vi "Serial Channel Output.vi"(0 "tagged llp packets cluster":T1, 1 "reset":bool, 2 "global counter":T25, 3 "common resources":T11={"sync pulse resources"={"sync pulse destination terminal"="", "sync100"="", "sync pulse source terminal"="", "imported sync pulse register"="", "generate sync pulse handshake"="", "enable sync pulse register"="", "sync pulse clock"=""}, "serial channel resources"={"sc 0"={"completed frames register"=""}, "sc 1"={"completed frames register"=""}, "sc 2"={"completed frames register"=""}, "sc 3"={"completed frames register"=""}, "sc 4"={"completed frames register"=""}, "sc 5"={"completed frames register"=""}, "sc 6"={"completed frames register"=""}, "sc 7"={"completed frames register"=""}}, "dram manager 0"={"DRAM class"=refnum, "process clock"="", "registers"={"configuration"={"write time slice"="", "request time slice"="", "DRAM arbiter config"="", "partition config"=""}, "reset"={"handshake"={"start.go"="", "start.go rcvd"="", "done.go"="", "done.go rcvd"=""}, "process"={"in"="", "out"=""}, "write"={"in"="", "out 0"="", "out 1"="", "out 2"="", "out 3"=""}, "read"={"in"="", "out 0"="", "out 1"="", "out 2"="", "out 3"=""}}, "status"={"partition full"=""}}, "FIFOs"={"write data"={"FIFO 0"="", "FIFO 1"="", "FIFO 2"="", "FIFO 3"=""}, "request metadata"={"FIFO"=""}, "read data VOQ"={"FIFO 0"="", "FIFO 1"="", "FIFO 2"="", "FIFO 3"=""}, "read data"={"FIFO 0"="", "FIFO 1"="", "FIFO 2"="", "FIFO 3"=""}}, "num active streams"=0.0, "max open read requests"=256}, "dram manager 1"={"DRAM class"=refnum, "process clock"="", "registers"={"configuration"={"write time slice"="", "request time slice"="", "DRAM arbiter config"="", "partition config"=""}, "reset"={"handshake"={"start.go"="", "start.go rcvd"="", "done.go"="", "done.go rcvd"=""}, "process"={"in"="", "out"=""}, "write"={"in"="", "out 0"="", "out 1"="", "out 2"="", "out 3"=""}, "read"={"in"="", "out 0"="", "out 1"="", "out 2"="", "out 3"=""}}, "status"={"partition full"=""}}, "FIFOs"={"write data"={"FIFO 0"="", "FIFO 1"="", "FIFO 2"="", "FIFO 3"=""}, "request metadata"={"FIFO"=""}, "read data VOQ"={"FIFO 0"="", "FIFO 1"="", "FIFO 2"="", "FIFO 3"=""}, "read data"={"FIFO 0"="", "FIFO 1"="", "FIFO 2"="", "FIFO 3"=""}}, "num active streams"=0.0, "max open read requests"=256}}, 5 "dram status":T22[](array[typedef]), 7 "start trigger":bool, 9 "output valid":bool[](array[boolean])=[FALSE, FALSE, FALSE, FALSE, FALSE, FALSE, FALSE, FALSE], 11 "stop trigger":bool, 12 "channel configs":T24[](array[typedef])) -> (4 "serial output channel status":T26[](array[typedef]), 6 "ready for start trigger":bool, 8 "packet timing error detected":bool, 10 "generation done":bool, 14 "ready for input":bool[](array[boolean]), 15 "i2c monitor array":T23[](array[typedef]) {"monitor word" format="%.0x"})   [LabVIEW 2020, in "GettingStarted_Gen_148X_FPGA.lvlib"]
uses:
  GettingStarted_Gen_148X_FPGA.lvlib
  Types/Serial Output Channel Status.ctl
  Common/Types/DRAM Status.ctl
  <instrlib>/FlexRIO/CSI-2/v2/FPGA/Types/Timestamp Counter Value.ctl
  Types/Serial Output Channel Datapath Configuration.ctl
  <instrlib>/FlexRIO/API/FPGA/v1/IO/NI148x/i2c monitor.ctl
  Common/Types/Common Resources.ctl
  <instrlib>/_niInstr/Memory/v1/FPGA/DRAM/niInstr Memory DRAM v1 FPGA.lvclass
  <instrlib>/FlexRIO/CSI-2/v2/FPGA/Types/Sync Pulse Resources.ctl
  Common/Types/Serial Channel Resources.ctl
  Common/Types/Single Serial Channel Resources.ctl
  <instrlib>/FlexRIO/CSI-2/v2/FPGA/DRAM Manager/Private/DRAM Manager.ctl
  <instrlib>/FlexRIO/CSI-2/v2/FPGA/DRAM Manager/Private/Common/DRAM Manager Registers.ctl
  <instrlib>/FlexRIO/CSI-2/v2/FPGA/DRAM Manager/Private/Common/Handshake Registers.ctl
  <instrlib>/FlexRIO/CSI-2/v2/FPGA/DRAM Manager/Private/Common/DRAM Manager FIFOs.ctl
  <instrlib>/FlexRIO/CSI-2/v2/FPGA/DRAM Manager/Private/Common/Write Data FIFO Ref.ctl
  <instrlib>/FlexRIO/CSI-2/v2/FPGA/DRAM Manager/Private/Common/Read Request Metadata FIFO Ref.ctl
  <instrlib>/FlexRIO/CSI-2/v2/FPGA/DRAM Manager/Private/Common/Read Data FIFO Ref.ctl
  Common/Types/Tagged LLP Packets Cluster.ctl
  <instrlib>/FlexRIO/CSI-2/v2/FPGA/Types/Tagged LLP Packet.ctl
  <instrlib>/FlexRIO/CSI-2/v2/FPGA/Types/FPGA LLP Packet Tag.ctl
  <instrlib>/FlexRIO/CSI-2/v2/FPGA/Types/FPGA LLP Packet Timestamp.ctl
  <instrlib>/FlexRIO/CSI-2/v2/FPGA/Types/Timestamp ID.ctl
  <instrlib>/FlexRIO/CSI-2/v2/FPGA/Types/FPGA LLP Packet Size.ctl
  <instrlib>/FlexRIO/CSI-2/v2/FPGA/Types/LLP Packet.ctl
  <instrlib>/FlexRIO/CSI-2/v2/FPGA/Types/LLP Packet Header.ctl
  <instrlib>/FlexRIO/CSI-2/v2/FPGA/Types/LLP Packet Payload.ctl
  <instrlib>/FlexRIO/CSI-2/v2/FPGA/Types/LLP Packet Footer.ctl
  Common/GettingStarted_Common_148X_FPGA.lvlib
  <instrlib>/_niInstr/Basic Elements/v1/FPGA/niInstr Basic Elements v1 FPGA.lvlib
  <instrlib>/FlexRIO/CSI-2/v2/FPGA/NI CSI-2 API FPGA v2.lvlib
  <instrlib>/FlexRIO/API/FPGA/v1/IO/NI148x/FlexRIO 148x FPGA v1.lvlib
  <instrlib>/FlexRIO/CSI-2/v2/FPGA/DRAM Manager/DRAM Manager v2.lvlib
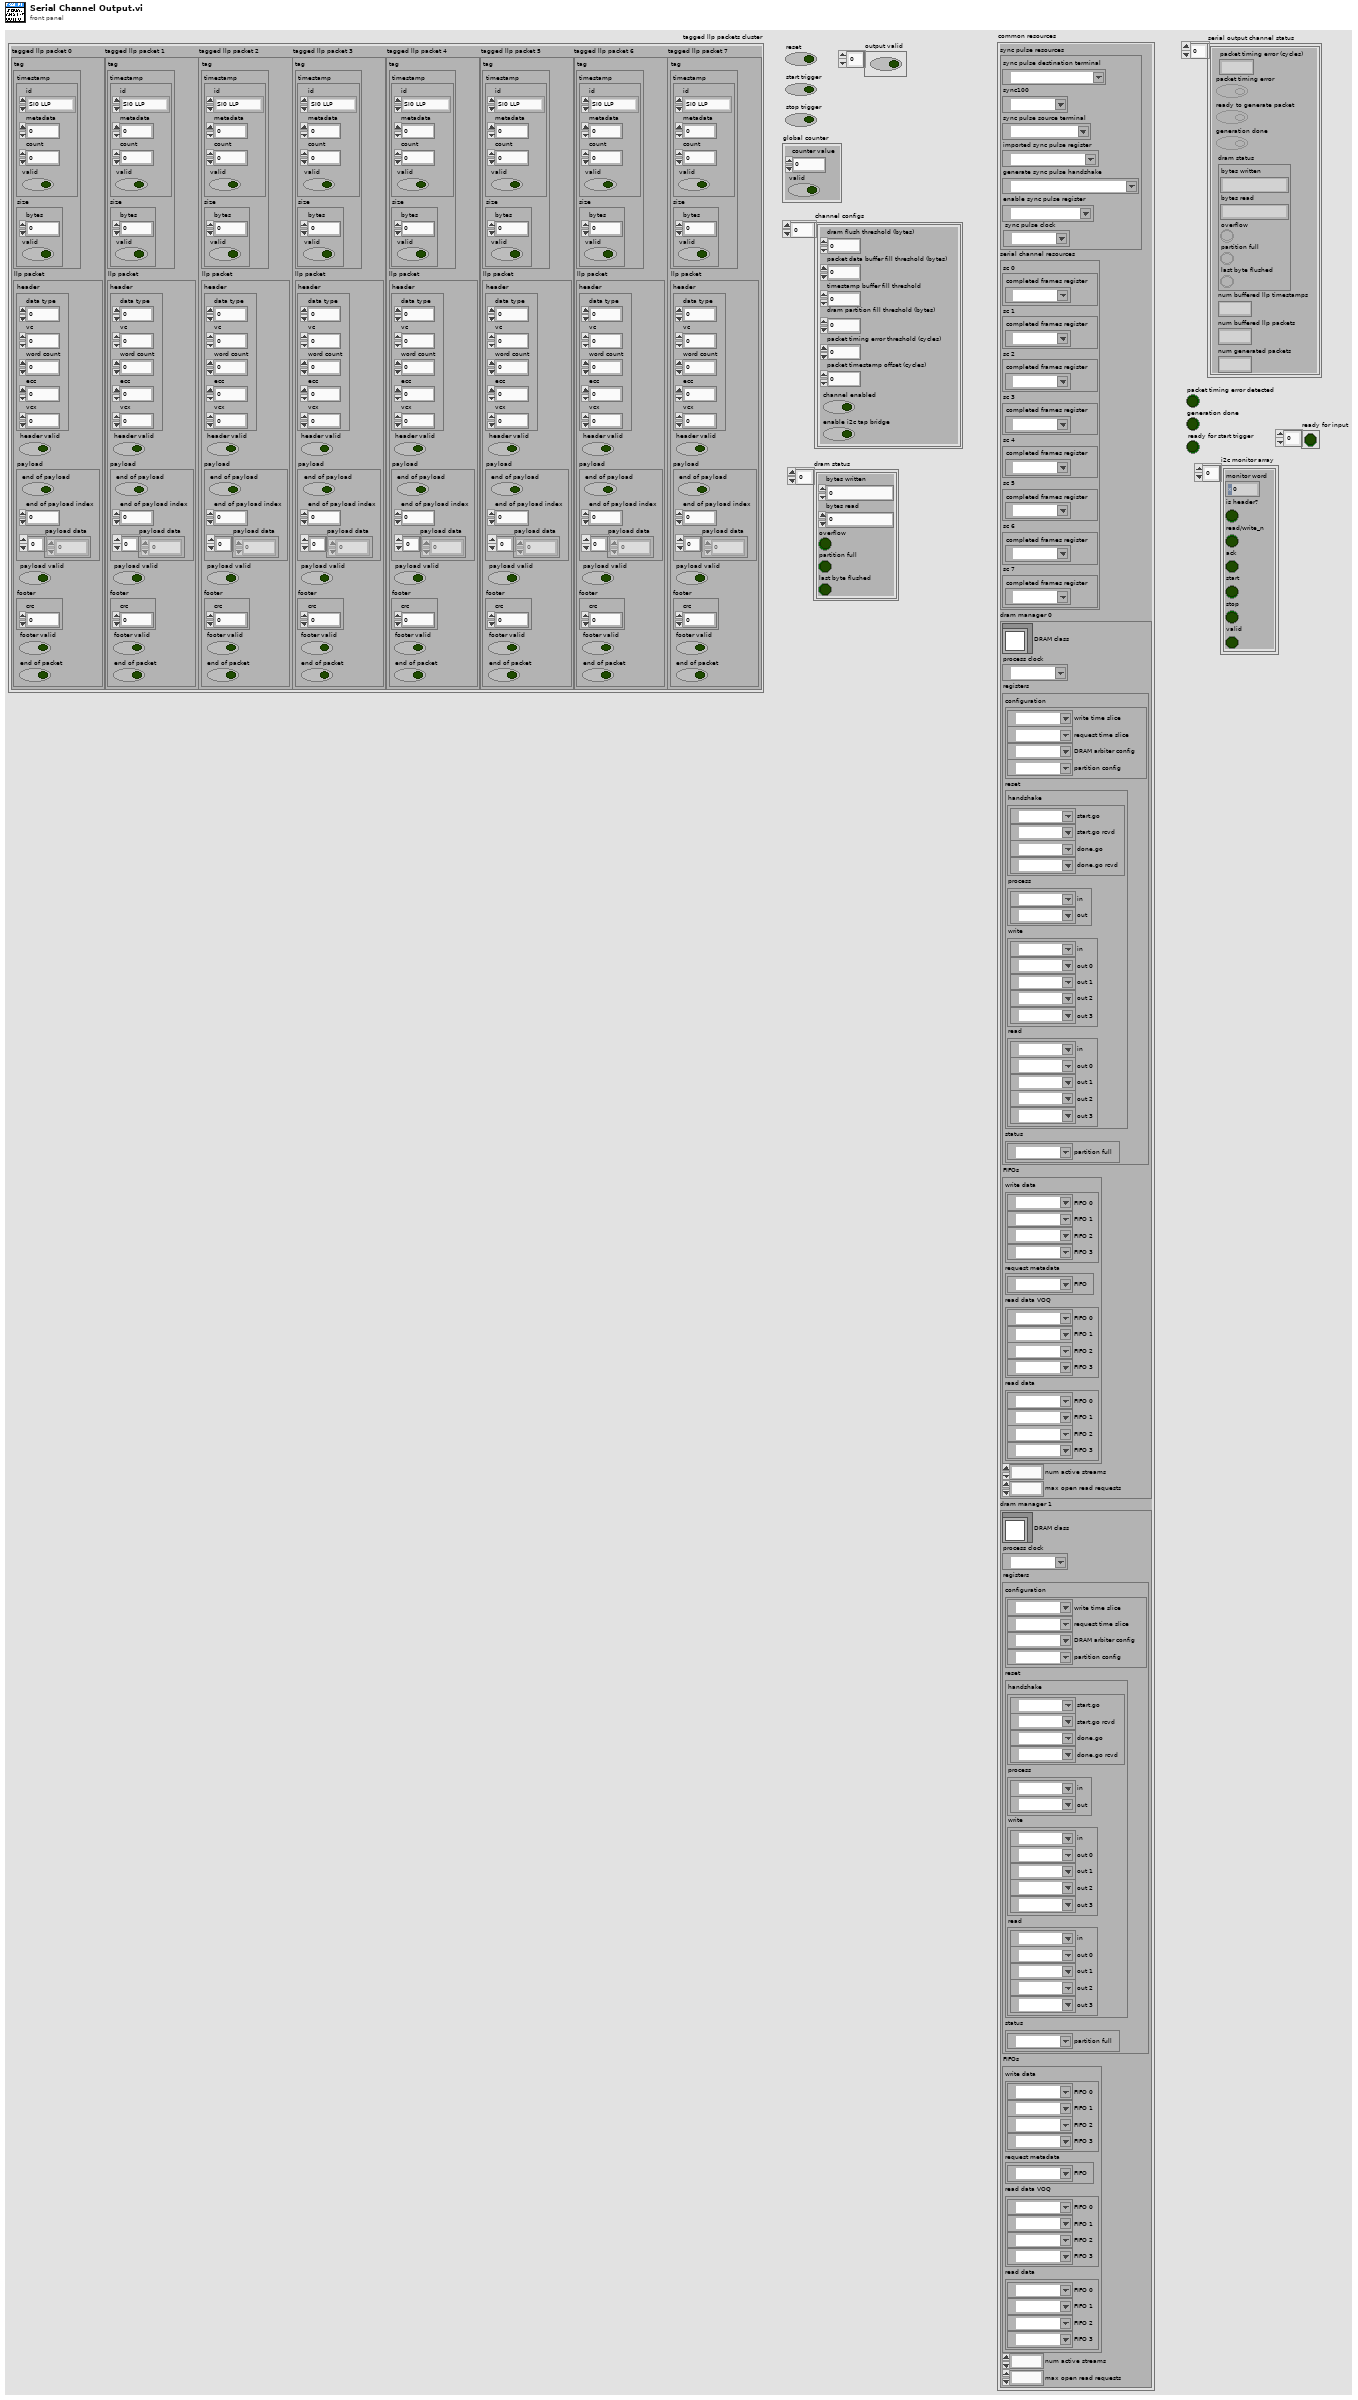
[diagram p1: front panel]
types:
  T1 = typedef "GettingStarted_Common_148X_FPGA.lvlib/Tagged LLP Packets Cluster.ctl" = cluster{"tagged llp packet 0":T2, "tagged llp packet 1":T2, "tagged llp packet 2":T2, "tagged llp packet 3":T2, "tagged llp packet 4":T2, "tagged llp packet 5":T2, "tagged llp packet 6":T2, "tagged llp packet 7":T2}
  T2 = typedef "NI CSI-2 API FPGA v2.lvlib/Tagged LLP Packet.ctl" = cluster{"tag":T3, "llp packet":T7}
  T3 = typedef "NI CSI-2 API FPGA v2.lvlib/FPGA LLP Packet Tag.ctl" = cluster{"timestamp":T4, "size":T6}
  T4 = typedef "NI CSI-2 API FPGA v2.lvlib/FPGA LLP Packet Timestamp.ctl" = cluster{"valid":bool, "count":fxp<+,50,50>, "id":T5, "metadata":u8}
  T5 = typedef "NI CSI-2 API FPGA v2.lvlib/Timestamp ID.ctl" = enum8{"SI0 LLP", "SI1 LLP", "SI2 LLP", "SI3 LLP", "SI4 LLP", "SI5 LLP", "SI6 LLP", "SI7 LLP", "SO0 LLP", "SO1 LLP", "SO2 LLP", "SO3 LLP", "SO4 LLP", "SO5 LLP", "SO6 LLP", "SO7 LLP", "Ser0 GPIO Bank", "Ser1 GPIO Bank", "Ser2 GPIO Bank", "Ser3 GPIO Bank", "Ser4 GPIO Bank", "Ser5 GPIO Bank", "Ser6 GPIO Bank", "Ser7 GPIO Bank", "Des0 GPIO Bank", "Des1 GPIO Bank", "Des2 GPIO Bank", "Des3 GPIO Bank", "Des4 GPIO Bank", "Des5 GPIO Bank", "Des6 GPIO Bank", "Des7 GPIO Bank", "User0", "User1", "User2", "User3", "User4", "User5", "User6", "User7", "User8", "User9", "User10", "User11", "User12", "User13", "User14", "User15", "User16", "User17", "User18", "User19", "User20", "User21", "User22", "User23", "User24", "User25", "User26", "User27", "User28", "User29", "User30", "User31"}
  T6 = typedef "NI CSI-2 API FPGA v2.lvlib/FPGA LLP Packet Size.ctl" = cluster{"bytes":fxp<+,17,17>, "valid":bool}
  T7 = typedef "NI CSI-2 API FPGA v2.lvlib/LLP Packet.ctl" = cluster{"header":T8, "header valid":bool, "payload":T9, "payload valid":bool, "footer":T10, "footer valid":bool, "end of packet":bool}
  T8 = typedef "NI CSI-2 API FPGA v2.lvlib/LLP Packet Header.ctl" = cluster{"word count":u16, "ecc":fxp<+,6,6>, "vcx":fxp<+,2,2>, "data type":fxp<+,6,6>, "vc":fxp<+,2,2>}
  T9 = typedef "NI CSI-2 API FPGA v2.lvlib/LLP Packet Payload.ctl" = cluster{"end of payload":bool, "end of payload index":fxp<+,3,3>, "payload data":u8[]}
  T10 = typedef "NI CSI-2 API FPGA v2.lvlib/LLP Packet Footer.ctl" = cluster{"crc":u16}
  T11 = typedef "GettingStarted_Common_148X_FPGA.lvlib/Common Resources.ctl" = cluster{"sync pulse resources":T12, "serial channel resources":T13, "dram manager 0":T15, "dram manager 1":T15}
  T12 = typedef "NI CSI-2 API FPGA v2.lvlib/Sync Pulse Resources.ctl" = cluster{"sync pulse destination terminal":refnum<k21>, "sync100":refnum<k21>, "sync pulse source terminal":refnum<k21>, "imported sync pulse register":refnum<k21>, "generate sync pulse handshake":refnum<k21>, "enable sync pulse register":refnum<k21>, "sync pulse clock":refnum<k21>}
  T13 = typedef "GettingStarted_Common_148X_FPGA.lvlib/Serial Channel Resources.ctl" = cluster{"sc 0":T14, "sc 1":T14, "sc 2":T14, "sc 3":T14, "sc 4":T14, "sc 5":T14, "sc 6":T14, "sc 7":T14}
  T14 = typedef "GettingStarted_Common_148X_FPGA.lvlib/Single Serial Channel Resources.ctl" = cluster{"completed frames register":refnum<k21>}
  T15 = typedef "DRAM Manager v2.lvlib/DRAM Manager.ctl" = cluster{"DRAM class":refnum<class "niInstr Memory DRAM v1 FPGA.lvclass">, "process clock":refnum<k21>, "registers":T16, "FIFOs":T18, "num active streams":fxp<+,3,3>, "max open read requests":u16}
  T16 = typedef "DRAM Manager v2.lvlib/DRAM Manager Registers.ctl" = cluster{"configuration":cluster{"write time slice":refnum<k21>, "request time slice":refnum<k21>, "DRAM arbiter config":refnum<k21>, "partition config":refnum<k21>}, "reset":cluster{"handshake":T17, "process":cluster{"in":refnum<k21>, "out":refnum<k21>}, "write":cluster{"in":refnum<k21>, "out 0":refnum<k21>, "out 1":refnum<k21>, "out 2":refnum<k21>, "out 3":refnum<k21>}, "read":cluster{"in":refnum<k21>, "out 0":refnum<k21>, "out 1":refnum<k21>, "out 2":refnum<k21>, "out 3":refnum<k21>}}, "status":cluster{"partition full":refnum<k21>}}
  T17 = typedef "DRAM Manager v2.lvlib/Handshake Registers.ctl" = cluster{"start.go":refnum<k21>, "start.go rcvd":refnum<k21>, "done.go":refnum<k21>, "done.go rcvd":refnum<k21>}
  T18 = typedef "DRAM Manager v2.lvlib/DRAM Manager FIFOs.ctl" = cluster{"write data":cluster{"FIFO 0":T19, "FIFO 1":T19, "FIFO 2":T19, "FIFO 3":T19}, "request metadata":cluster{"FIFO":T20}, "read data VOQ":cluster{"FIFO 0":T21, "FIFO 1":T21, "FIFO 2":T21, "FIFO 3":T21}, "read data":cluster{"FIFO 0":T21, "FIFO 1":T21, "FIFO 2":T21, "FIFO 3":T21}}
  T19 = typedef "DRAM Manager v2.lvlib/Write Data FIFO Ref.ctl" = refnum<k21>
  T20 = typedef "DRAM Manager v2.lvlib/Read Request Metadata FIFO Ref.ctl" = refnum<k21>
  T21 = typedef "DRAM Manager v2.lvlib/Read Data FIFO Ref.ctl" = refnum<k21>
  T22 = typedef "GettingStarted_Common_148X_FPGA.lvlib/DRAM Status.ctl" = cluster{"bytes written":u64, "bytes read":u64, "overflow":bool, "partition full":bool, "last byte flushed":bool}
  T23 = typedef "FlexRIO 148x FPGA v1.lvlib/i2c monitor.ctl" = cluster{"monitor word":u8, "is header?":bool, "read/write_n":bool, "ack":bool, "start":bool, "stop":bool, "valid":bool}
  T24 = typedef "GettingStarted_Gen_148X_FPGA.lvlib/Serial Output Channel Datapath Configuration.ctl" = cluster{"dram flush threshold (bytes)":u64, "packet data buffer fill threshold (bytes)":u64, "timestamp buffer fill threshold":u32, "packet timing error threshold (cycles)":u64, "channel enabled":bool, "dram partition fill threshold (bytes)":u64, "enable i2c tap bridge":bool, "packet timestamp offset (cycles)":i64}
  T25 = typedef "NI CSI-2 API FPGA v2.lvlib/Timestamp Counter Value.ctl" = cluster{"counter value":u64, "valid":bool}
  T26 = typedef "GettingStarted_Gen_148X_FPGA.lvlib/Serial Output Channel Status.ctl" = cluster{"num buffered llp packets":fxp<+,14,14>, "packet timing error (cycles)":u64, "packet timing error":bool, "ready to generate packet":bool, "dram status":T22, "num buffered llp timestamps":u32, "generation done":bool, "num generated packets":u64}
  T27 = cluster{"datapath configs":T24, "tagged llp packet":T2, "output valid":bool, "dram status":T22}
  T28 = typedef "GettingStarted_Gen_148X_FPGA.lvlib/8 Out Channel Resources.ctl" = cluster{"so 0 resources":T29, "so 1 resources":T29, "so 2 resources":T29, "so 3 resources":T29, "so 4 resources":T29, "so 5 resources":T29, "so 6 resources":T29, "so 7 resources":T29}
  T29 = typedef "GettingStarted_Gen_148X_FPGA.lvlib/Serial Output Channel Resources.ctl" = cluster{"csi-2 output io":T30, "serial output channel instance":u8, "i2c io":T31, "sc resources":T14}
  T30 = typedef "GettingStarted_Common_148X_FPGA.lvlib/Serial Output Channel IO.ctl" = cluster{"csi-2 axi stream tdata":refnum<k21>, "csi-2 axi stream tlast":refnum<k21>, "csi-2 axi stream tvalid":refnum<k21>, "csi-2 axi stream tuser":refnum<k21>, "csi-2 axi stream tready":refnum<k21>, "num packets in tx fifo":refnum<k21>, "ready to transmit packet":refnum<k21>, "transmit packet done":refnum<k21>, "transmit packet":refnum<k21>}
  T31 = typedef "GettingStarted_Common_148X_FPGA.lvlib/I2C IO.ctl" = cluster{"sda input":refnum<k21>, "sda output enable":refnum<k21>, "scl input":refnum<k21>, "scl output enable":refnum<k21>}
  T32 = typedef "GettingStarted_Gen_148X_FPGA.lvlib/4 In 4 Out Channel Resources.ctl" = cluster{"so 0 resources":T29, "so 1 resources":T29, "so 2 resources":T29, "so 3 resources":T29, "si 0 resources":T33, "si 1 resources":T33, "si 2 resources":T33, "si 3 resources":T33}
  T33 = typedef "GettingStarted_Gen_148X_FPGA.lvlib/Serial Input Channel Resources.ctl" = cluster{"i2c io":T31}
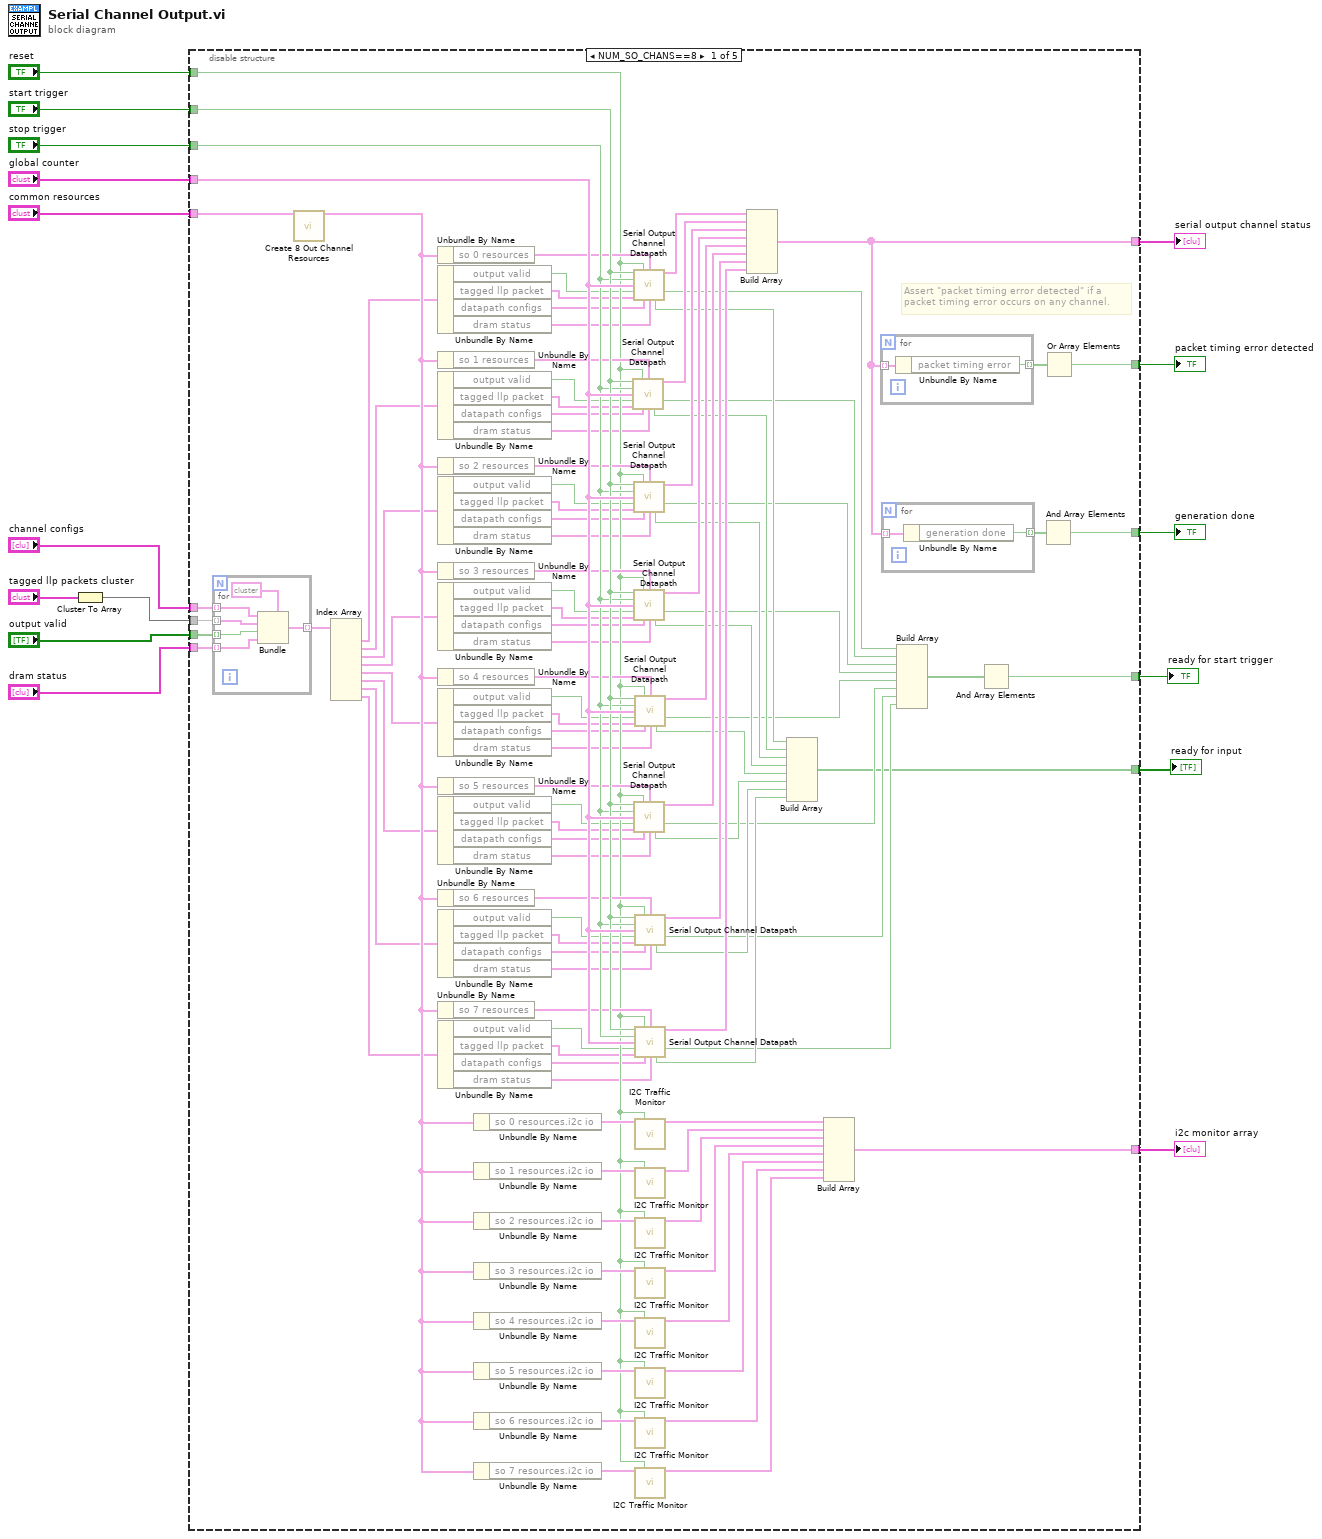
[diagram p0: block diagram]
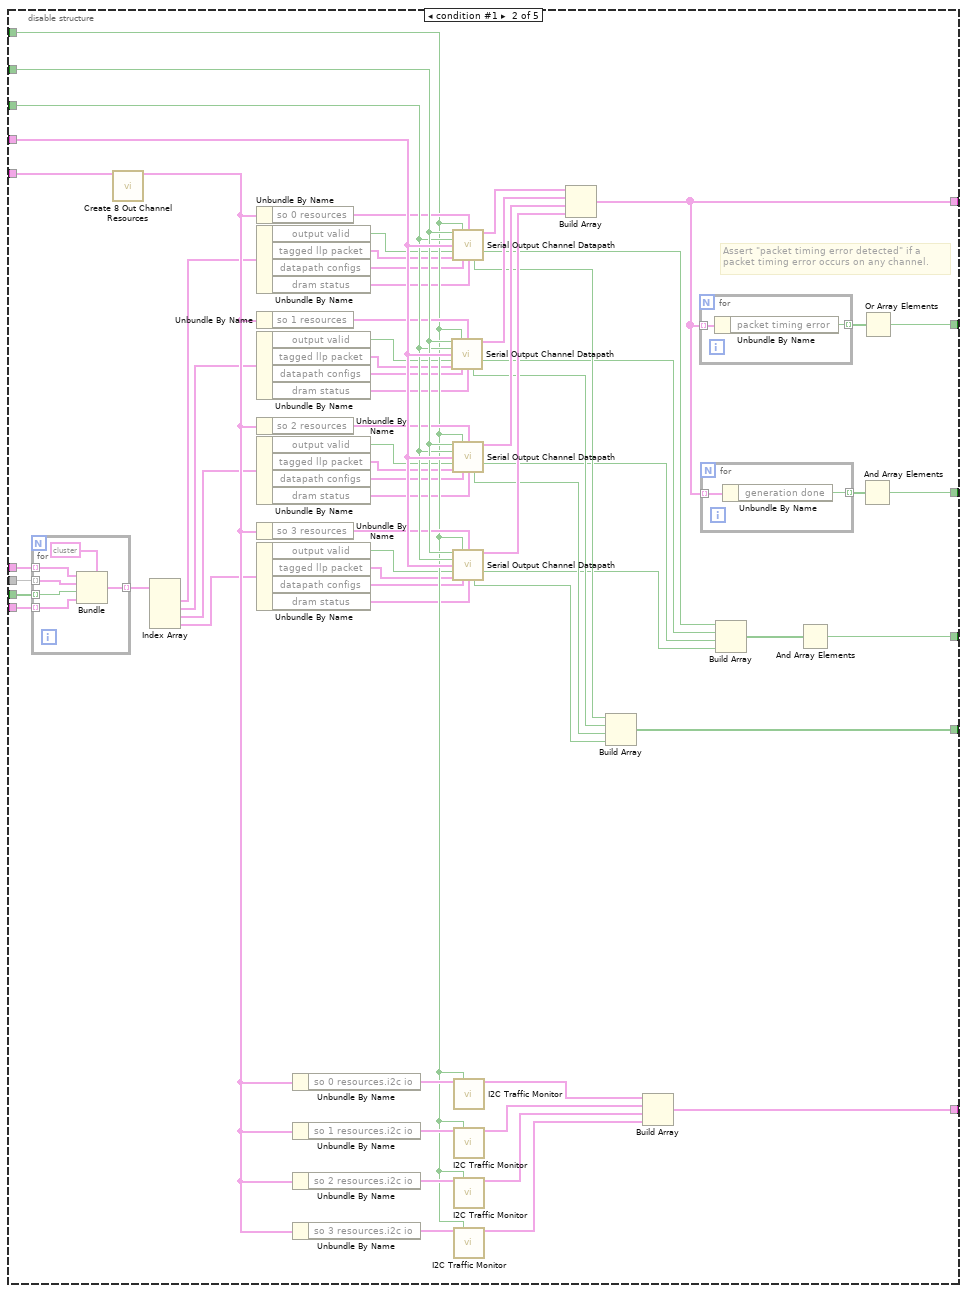
[diagram p2: hidden frame]
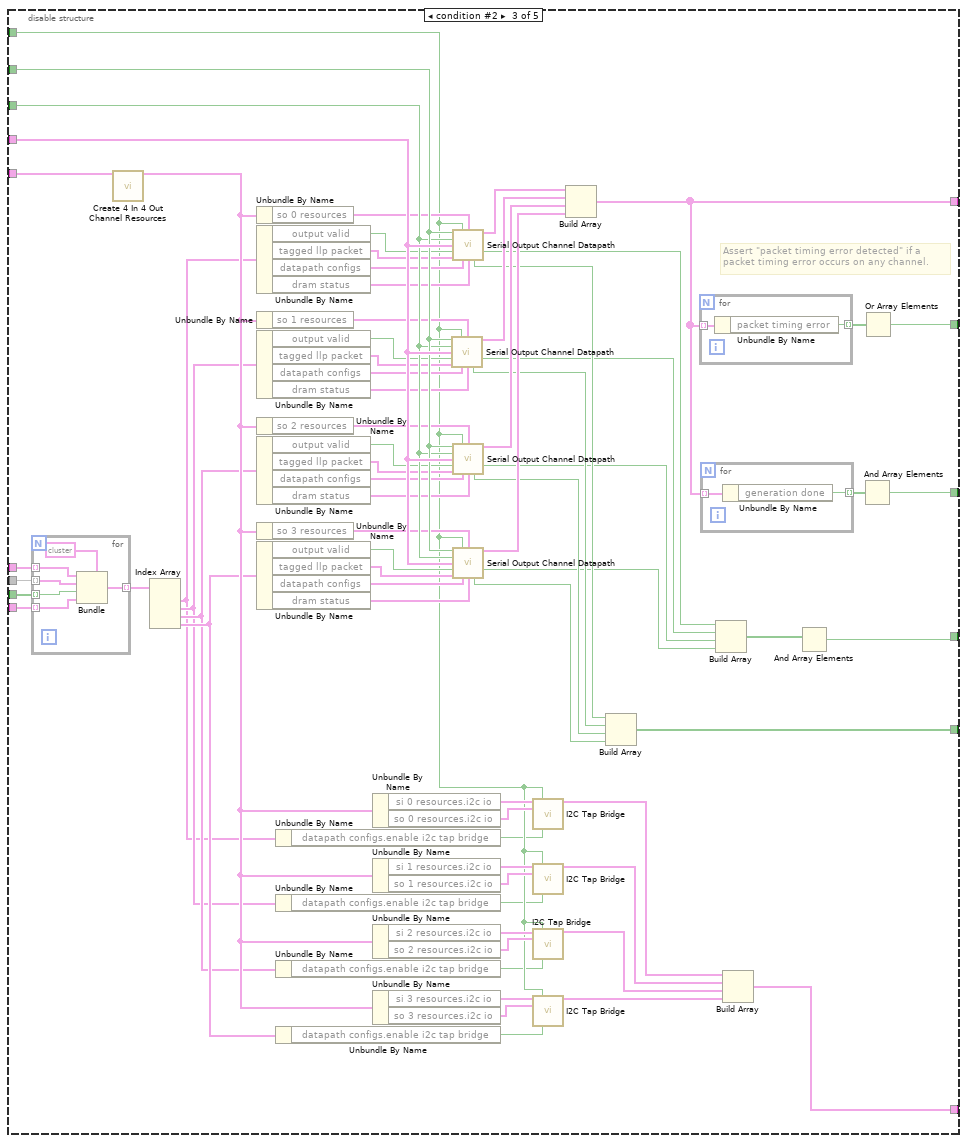
[diagram p3: hidden frame]
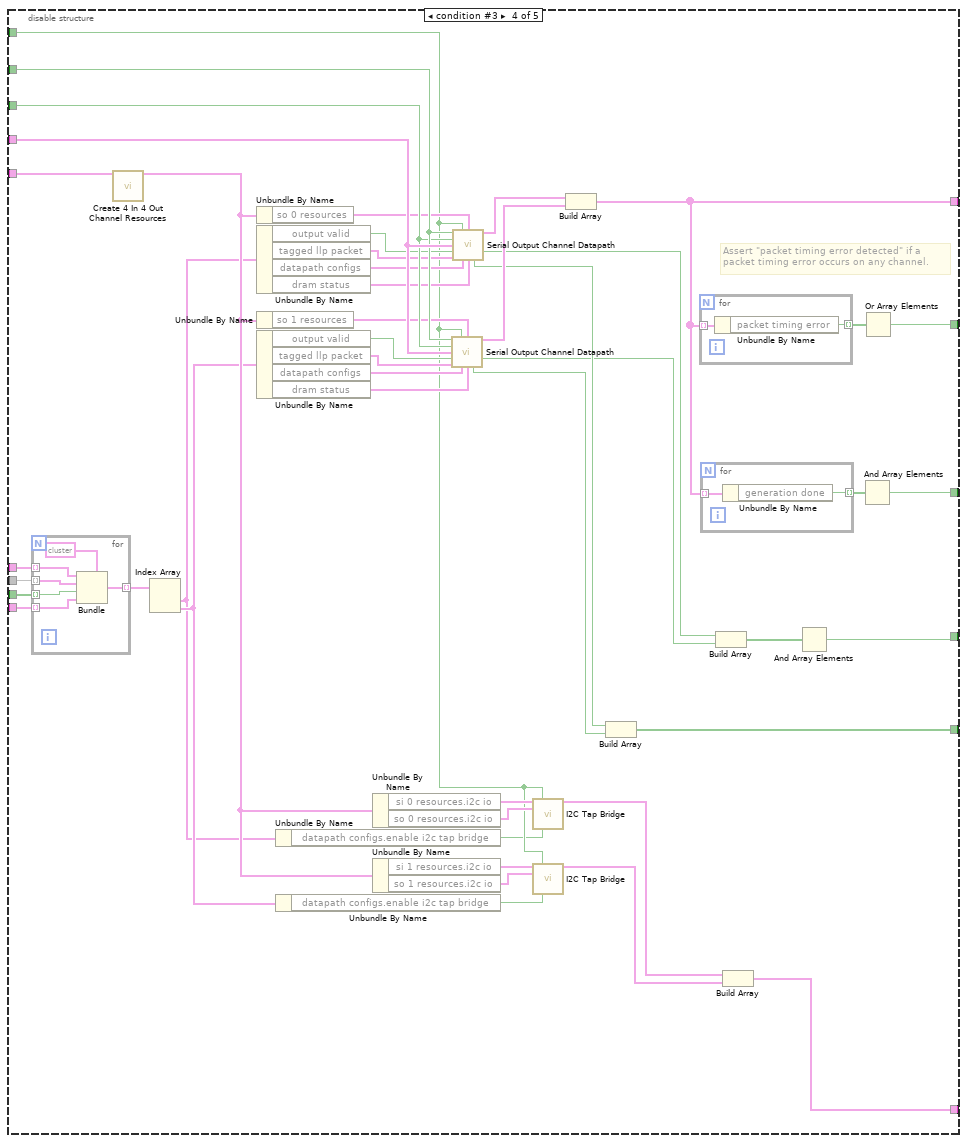
[diagram p4: hidden frame]
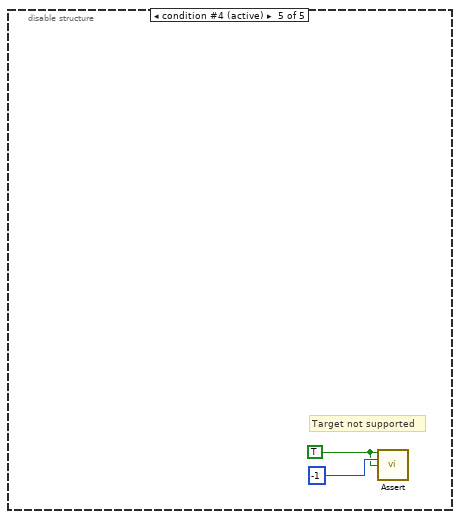
[diagram p5: hidden frame]
diagram:
  n1 = Cluster To Array(cluster="tagged llp packets cluster") -> (array=w1:T2[])
  n2 = disable-structure shown="NUM_SO_CHANS==8" {
    disable-tunnel: "global counter" -> [w124 w198 w280 w336 _]
    disable-tunnel: "start trigger" -> [w123 w197 w279 w335 _]
    disable-tunnel: "stop trigger" -> [w122 w196 w278 w334 _]
    disable-tunnel: [w98 w182 w264 w326 _] -> w13
    disable-tunnel: [w97 w181 w263 w325 _] -> w12
    disable-tunnel: [w95 w179 w261 w323 _] -> w11
    disable-tunnel: [w92 w176 w260 w322 _] -> w10
    disable-tunnel: "reset" -> [w77 w169 w216 w295 _]
    disable-tunnel: "channel configs" -> [w75 w167 w258 w320 _]
    disable-tunnel: w1 -> [w74 w166 w257 w319 _]
    disable-tunnel: "output valid" -> [w73 w165 w256 w318 _]
    disable-tunnel: "dram status" -> [w72 w164 w255 w317 _]
    disable-tunnel: [w18 w136 w231 w303 _] -> w4
    disable-tunnel: "common resources" -> [w20 w138 w233 w305 _]
    disable-tunnel: [w17 w135 w230 w302 _] -> w3
    frame condition #0 {
      # "Assert \"packet timing error detected\" if a \npacket timing error occurs on any channel."
      n3 = for {
        tunnel: w75 -> [w130] mode=indexing
        tunnel: w74 -> [w127] mode=indexing
        tunnel: w73 -> [w128] mode=indexing
        tunnel: w72 -> [w129] mode=indexing
        tunnel: [w126] -> w71 mode=indexing
        n4 = Bundle(cluster=T27 {"datapath configs"={"dram flush threshold (bytes)"=0, "packet data buffer fill threshold (bytes)"=0, "timestamp buffer fill threshold"=0, "packet timing error threshold (cycles)"=0, "channel enabled"=FALSE, "dram partition fill threshold (bytes)"=0, "enable i2c tap bridge"=FALSE, "packet timestamp offset (cycles)"=0}, "tagged llp packet"={"tag"={"timestamp"={"valid"=FALSE, "count"=0.0, "id"=enum."SI0 LLP", "metadata"=0}, "size"={"bytes"=0.0, "valid"=FALSE}}, "llp packet"={"header"={"word count"=0, "ecc"=0.0, "vcx"=0.0, "data type"=0.0, "vc"=0.0}, "header valid"=FALSE, "payload"={"end of payload"=FALSE, "end of payload index"=0.0, "payload data"=[]}, "payload valid"=FALSE, "footer"={"crc"=0}, "footer valid"=FALSE, "end of packet"=FALSE}}, "output valid"=FALSE, "dram status"={"bytes written"=0, "bytes read"=0, "overflow"=FALSE, "partition full"=FALSE, "last byte flushed"=FALSE}} ("element"), "datapath configs"=w130, "tagged llp packet"=w127, "output valid"=w128, "dram status"=w129) -> (w126:T27)
      }
      n5 = call "Create 8 Out Channel Resources.vi"("common resources"=w20) -> ("channel resources"=w76:T28)  [unwired: 14 in]
      n6 = Index Array(array=w71) -> (element #1=w70:T27, element #2=w67:T27, element #3=w66:T27, element #4=w64:T27, element #5=w63:T27, element #6=w65:T27, element #7=w68:T27, element #8=w69:T27)  [unwired: 8 in]
      n7 = Unbundle By Name(w76) -> ("so 0 resources"=w105:T29)
      n8 = Unbundle By Name(w70) -> ("output valid"=w62:bool, "tagged llp packet"=w61:T2, "datapath configs"=w60:T24, "dram status"=w59:T22)
      n9 = Unbundle By Name(w76) -> ("so 1 resources"=w106:T29)
      n10 = Unbundle By Name(w67) -> ("output valid"=w52:bool, "tagged llp packet"=w51:T2, "datapath configs"=w57:T24, "dram status"=w58:T22)
      n11 = Unbundle By Name(w76) -> ("so 2 resources"=w109:T29)
      n12 = Unbundle By Name(w66) -> ("output valid"=w54:bool, "tagged llp packet"=w53:T2, "datapath configs"=w56:T24, "dram status"=w55:T22)
      n13 = Unbundle By Name(w76) -> ("so 3 resources"=w108:T29)
      n14 = Unbundle By Name(w64) -> ("output valid"=w50:bool, "tagged llp packet"=w49:T2, "datapath configs"=w48:T24, "dram status"=w47:T22)
      n15 = Unbundle By Name(w76) -> ("so 4 resources"=w100:T29)
      n16 = Unbundle By Name(w63) -> ("output valid"=w43:bool, "tagged llp packet"=w44:T2, "datapath configs"=w45:T24, "dram status"=w46:T22)
      n17 = Unbundle By Name(w76) -> ("so 5 resources"=w101:T29)
      n18 = Unbundle By Name(w65) -> ("output valid"=w39:bool, "tagged llp packet"=w40:T2, "datapath configs"=w42:T24, "dram status"=w41:T22)
      n19 = Unbundle By Name(w76) -> ("so 6 resources"=w103:T29)
      n20 = Unbundle By Name(w68) -> ("output valid"=w35:bool, "tagged llp packet"=w36:T2, "datapath configs"=w38:T24, "dram status"=w37:T22)
      n21 = Unbundle By Name(w76) -> ("so 7 resources"=w102:T29)
      n22 = Unbundle By Name(w69) -> ("output valid"=w31:bool, "tagged llp packet"=w32:T2, "datapath configs"=w33:T24, "dram status"=w34:T22)
      n23 = Unbundle By Name(w76) -> ("so 0 resources.i2c io"=w94:T31)
      n24 = Unbundle By Name(w76) -> ("so 1 resources.i2c io"=w91:T31)
      n25 = Unbundle By Name(w76) -> ("so 2 resources.i2c io"=w90:T31)
      n26 = Unbundle By Name(w76) -> ("so 3 resources.i2c io"=w89:T31)
      n27 = Unbundle By Name(w76) -> ("so 4 resources.i2c io"=w88:T31)
      n28 = Unbundle By Name(w76) -> ("so 5 resources.i2c io"=w87:T31)
      n29 = Unbundle By Name(w76) -> ("so 6 resources.i2c io"=w86:T31)
      n30 = Unbundle By Name(w76) -> ("so 7 resources.i2c io"=w85:T31)
      n31 = call "Serial Output Channel Datapath.vi"("start trigger"=w123, "reset"=w77, "resources"=w106, "stop trigger"=w122, "generation counter"=w124, "output valid"=w52, "tagged llp packet"=w51, "configuration"=w57, "dram status"=w58) -> ("channel status"=w115:T26, "ready for start trigger"=w29:bool, "ready for input"=w107:bool)  [unwired: 4 in]
      n32 = call "Serial Output Channel Datapath.vi"("start trigger"=w123, "reset"=w77, "resources"=w105, "stop trigger"=w122, "generation counter"=w124, "output valid"=w62, "tagged llp packet"=w61, "configuration"=w60, "dram status"=w59) -> ("channel status"=w114:T26, "ready for start trigger"=w30:bool, "ready for input"=w104:bool)  [unwired: 4 in]
      n33 = call "Serial Output Channel Datapath.vi"("start trigger"=w123, "reset"=w77, "resources"=w109, "stop trigger"=w122, "generation counter"=w124, "output valid"=w54, "tagged llp packet"=w53, "configuration"=w56, "dram status"=w55) -> ("channel status"=w116:T26, "ready for start trigger"=w28:bool, "ready for input"=w110:bool)  [unwired: 4 in]
      n34 = call "Serial Output Channel Datapath.vi"("start trigger"=w123, "reset"=w77, "resources"=w108, "stop trigger"=w122, "generation counter"=w124, "output valid"=w50, "tagged llp packet"=w49, "configuration"=w48, "dram status"=w47) -> ("channel status"=w117:T26, "ready for start trigger"=w27:bool, "ready for input"=w111:bool)  [unwired: 4 in]
      n35 = call "Serial Output Channel Datapath.vi"("start trigger"=w123, "reset"=w77, "resources"=w101, "stop trigger"=w122, "generation counter"=w124, "output valid"=w39, "tagged llp packet"=w40, "configuration"=w42, "dram status"=w41) -> ("channel status"=w119:T26, "ready for start trigger"=w23:bool, "ready for input"=w26:bool)  [unwired: 4 in]
      n36 = call "Serial Output Channel Datapath.vi"("start trigger"=w123, "reset"=w77, "resources"=w100, "stop trigger"=w122, "generation counter"=w124, "output valid"=w43, "tagged llp packet"=w44, "configuration"=w45, "dram status"=w46) -> ("channel status"=w118:T26, "ready for start trigger"=w24:bool, "ready for input"=w112:bool)  [unwired: 4 in]
      n37 = call "Serial Output Channel Datapath.vi"("start trigger"=w123, "reset"=w77, "resources"=w103, "stop trigger"=w122, "generation counter"=w124, "output valid"=w35, "tagged llp packet"=w36, "configuration"=w38, "dram status"=w37) -> ("channel status"=w120:T26, "ready for start trigger"=w22:bool, "ready for input"=w25:bool)  [unwired: 4 in]
      n38 = call "Serial Output Channel Datapath.vi"("start trigger"=w123, "reset"=w77, "resources"=w102, "stop trigger"=w122, "generation counter"=w124, "output valid"=w31, "tagged llp packet"=w32, "configuration"=w33, "dram status"=w34) -> ("channel status"=w121:T26, "ready for start trigger"=w21:bool, "ready for input"=w113:bool)  [unwired: 4 in]
      n39 = call "I2C Traffic Monitor.vi"("channel i2c io"=w94, "reset"=w77) -> ("i2c monitor"=w93:T23)  [unwired: 13 in]
      n40 = call "I2C Traffic Monitor.vi"("channel i2c io"=w91, "reset"=w77) -> ("i2c monitor"=w84:T23)  [unwired: 13 in]
      n41 = call "I2C Traffic Monitor.vi"("channel i2c io"=w90, "reset"=w77) -> ("i2c monitor"=w83:T23)  [unwired: 13 in]
      n42 = call "I2C Traffic Monitor.vi"("channel i2c io"=w89, "reset"=w77) -> ("i2c monitor"=w82:T23)  [unwired: 13 in]
      n43 = call "I2C Traffic Monitor.vi"("channel i2c io"=w88, "reset"=w77) -> ("i2c monitor"=w81:T23)  [unwired: 13 in]
      n44 = call "I2C Traffic Monitor.vi"("channel i2c io"=w87, "reset"=w77) -> ("i2c monitor"=w80:T23)  [unwired: 13 in]
      n45 = call "I2C Traffic Monitor.vi"("channel i2c io"=w86, "reset"=w77) -> ("i2c monitor"=w79:T23)  [unwired: 13 in]
      n46 = call "I2C Traffic Monitor.vi"("channel i2c io"=w85, "reset"=w77) -> ("i2c monitor"=w78:T23)  [unwired: 13 in]
      n47 = Build Array(w114, w115, w116, w117, w118, w119, w120, w121) -> (w97:T26[])
      n48 = Build Array(w104, w107, w110, w111, w112, w26, w25, w113) -> (w17:bool[])
      n49 = Build Array(w93, w84, w83, w82, w81, w80, w79, w78) -> (w92:T23[])
      n50 = for {
        tunnel: w97 -> [w134] mode=indexing
        tunnel: [w133] -> w99 mode=indexing
        n51 = Unbundle By Name(w134) -> ("packet timing error"=w133:bool)
      }
      n52 = for {
        tunnel: w97 -> [w132] mode=indexing
        tunnel: [w131] -> w96 mode=indexing
        n53 = Unbundle By Name(w132) -> ("generation done"=w131:bool)
      }
      n54 = Build Array(w30, w29, w28, w27, w24, w23, w22, w21) -> (w19:bool[])
      n55 = And Array Elements(Boolean array=w19) -> (logical AND=w18:bool)
      n56 = And Array Elements(Boolean array=w96) -> (logical AND=w95:bool)
      n57 = Or Array Elements(Boolean array=w99) -> (logical OR=w98:bool)
    }
    frame condition #1 {
      # "Assert \"packet timing error detected\" if a \npacket timing error occurs on any channel."
      n58 = for {
        tunnel: w167 -> [w204] mode=indexing
        tunnel: w166 -> [w201] mode=indexing
        tunnel: w165 -> [w202] mode=indexing
        tunnel: w164 -> [w203] mode=indexing
        tunnel: [w200] -> w163 mode=indexing
        n59 = Bundle(cluster=T27 {"datapath configs"={"dram flush threshold (bytes)"=0, "packet data buffer fill threshold (bytes)"=0, "timestamp buffer fill threshold"=0, "packet timing error threshold (cycles)"=0, "channel enabled"=FALSE, "dram partition fill threshold (bytes)"=0, "enable i2c tap bridge"=FALSE, "packet timestamp offset (cycles)"=0}, "tagged llp packet"={"tag"={"timestamp"={"valid"=FALSE, "count"=0.0, "id"=enum."SI0 LLP", "metadata"=0}, "size"={"bytes"=0.0, "valid"=FALSE}}, "llp packet"={"header"={"word count"=0, "ecc"=0.0, "vcx"=0.0, "data type"=0.0, "vc"=0.0}, "header valid"=FALSE, "payload"={"end of payload"=FALSE, "end of payload index"=0.0, "payload data"=[]}, "payload valid"=FALSE, "footer"={"crc"=0}, "footer valid"=FALSE, "end of packet"=FALSE}}, "output valid"=FALSE, "dram status"={"bytes written"=0, "bytes read"=0, "overflow"=FALSE, "partition full"=FALSE, "last byte flushed"=FALSE}} ("element"), "datapath configs"=w204, "tagged llp packet"=w201, "output valid"=w202, "dram status"=w203) -> (w200:T27)
      }
      n60 = call "Create 8 Out Channel Resources.vi"("common resources"=w138) -> ("channel resources"=w168:T28)  [unwired: 14 in]
      n61 = Index Array(array=w163) -> (element #1=w162:T27, element #2=w161:T27, element #3=w160:T27, element #4=w159:T27)  [unwired: 4 in]
      n62 = Unbundle By Name(w168) -> ("so 0 resources"=w185:T29)
      n63 = Unbundle By Name(w162) -> ("output valid"=w158:bool, "tagged llp packet"=w157:T2, "datapath configs"=w156:T24, "dram status"=w155:T22)
      n64 = Unbundle By Name(w168) -> ("so 1 resources"=w186:T29)
      n65 = Unbundle By Name(w161) -> ("output valid"=w148:bool, "tagged llp packet"=w147:T2, "datapath configs"=w153:T24, "dram status"=w154:T22)
      n66 = Unbundle By Name(w168) -> ("so 2 resources"=w189:T29)
      n67 = Unbundle By Name(w160) -> ("output valid"=w150:bool, "tagged llp packet"=w149:T2, "datapath configs"=w152:T24, "dram status"=w151:T22)
      n68 = Unbundle By Name(w168) -> ("so 3 resources"=w188:T29)
      n69 = Unbundle By Name(w159) -> ("output valid"=w146:bool, "tagged llp packet"=w145:T2, "datapath configs"=w144:T24, "dram status"=w143:T22)
      n70 = Unbundle By Name(w168) -> ("so 0 resources.i2c io"=w178:T31)
      n71 = Unbundle By Name(w168) -> ("so 1 resources.i2c io"=w175:T31)
      n72 = Unbundle By Name(w168) -> ("so 2 resources.i2c io"=w174:T31)
      n73 = Unbundle By Name(w168) -> ("so 3 resources.i2c io"=w173:T31)
      n74 = call "Serial Output Channel Datapath.vi"("start trigger"=w197, "reset"=w169, "resources"=w186, "stop trigger"=w196, "generation counter"=w198, "output valid"=w148, "tagged llp packet"=w147, "configuration"=w153, "dram status"=w154) -> ("channel status"=w193:T26, "ready for start trigger"=w141:bool, "ready for input"=w187:bool)  [unwired: 4 in]
      n75 = call "Serial Output Channel Datapath.vi"("start trigger"=w197, "reset"=w169, "resources"=w185, "stop trigger"=w196, "generation counter"=w198, "output valid"=w158, "tagged llp packet"=w157, "configuration"=w156, "dram status"=w155) -> ("channel status"=w192:T26, "ready for start trigger"=w142:bool, "ready for input"=w184:bool)  [unwired: 4 in]
      n76 = call "Serial Output Channel Datapath.vi"("start trigger"=w197, "reset"=w169, "resources"=w189, "stop trigger"=w196, "generation counter"=w198, "output valid"=w150, "tagged llp packet"=w149, "configuration"=w152, "dram status"=w151) -> ("channel status"=w194:T26, "ready for start trigger"=w140:bool, "ready for input"=w190:bool)  [unwired: 4 in]
      n77 = call "Serial Output Channel Datapath.vi"("start trigger"=w197, "reset"=w169, "resources"=w188, "stop trigger"=w196, "generation counter"=w198, "output valid"=w146, "tagged llp packet"=w145, "configuration"=w144, "dram status"=w143) -> ("channel status"=w195:T26, "ready for start trigger"=w139:bool, "ready for input"=w191:bool)  [unwired: 4 in]
      n78 = call "I2C Traffic Monitor.vi"("channel i2c io"=w178, "reset"=w169) -> ("i2c monitor"=w177:T23)  [unwired: 13 in]
      n79 = call "I2C Traffic Monitor.vi"("channel i2c io"=w175, "reset"=w169) -> ("i2c monitor"=w172:T23)  [unwired: 13 in]
      n80 = call "I2C Traffic Monitor.vi"("channel i2c io"=w174, "reset"=w169) -> ("i2c monitor"=w171:T23)  [unwired: 13 in]
      n81 = call "I2C Traffic Monitor.vi"("channel i2c io"=w173, "reset"=w169) -> ("i2c monitor"=w170:T23)  [unwired: 13 in]
      n82 = Build Array(w192, w193, w194, w195) -> (w181:T26[])
      n83 = Build Array(w184, w187, w190, w191) -> (w135:bool[])
      n84 = Build Array(w177, w172, w171, w170) -> (w176:T23[])
      n85 = for {
        tunnel: w181 -> [w208] mode=indexing
        tunnel: [w207] -> w183 mode=indexing
        n86 = Unbundle By Name(w208) -> ("packet timing error"=w207:bool)
      }
      n87 = for {
        tunnel: w181 -> [w206] mode=indexing
        tunnel: [w205] -> w180 mode=indexing
        n88 = Unbundle By Name(w206) -> ("generation done"=w205:bool)
      }
      n89 = Build Array(w142, w141, w140, w139) -> (w137:bool[])
      n90 = And Array Elements(Boolean array=w137) -> (logical AND=w136:bool)
      n91 = And Array Elements(Boolean array=w180) -> (logical AND=w179:bool)
      n92 = Or Array Elements(Boolean array=w183) -> (logical OR=w182:bool)
    }
    frame condition #2 {
      # "Assert \"packet timing error detected\" if a \npacket timing error occurs on any channel."
      n93 = for {
        tunnel: w258 -> [w286] mode=indexing
        tunnel: w257 -> [w283] mode=indexing
        tunnel: w256 -> [w284] mode=indexing
        tunnel: w255 -> [w285] mode=indexing
        tunnel: [w282] -> w254 mode=indexing
        n94 = Bundle(cluster=T27 {"datapath configs"={"dram flush threshold (bytes)"=0, "packet data buffer fill threshold (bytes)"=0, "timestamp buffer fill threshold"=0, "packet timing error threshold (cycles)"=0, "channel enabled"=FALSE, "dram partition fill threshold (bytes)"=0, "enable i2c tap bridge"=FALSE, "packet timestamp offset (cycles)"=0}, "tagged llp packet"={"tag"={"timestamp"={"valid"=FALSE, "count"=0.0, "id"=enum."SI0 LLP", "metadata"=0}, "size"={"bytes"=0.0, "valid"=FALSE}}, "llp packet"={"header"={"word count"=0, "ecc"=0.0, "vcx"=0.0, "data type"=0.0, "vc"=0.0}, "header valid"=FALSE, "payload"={"end of payload"=FALSE, "end of payload index"=0.0, "payload data"=[]}, "payload valid"=FALSE, "footer"={"crc"=0}, "footer valid"=FALSE, "end of packet"=FALSE}}, "output valid"=FALSE, "dram status"={"bytes written"=0, "bytes read"=0, "overflow"=FALSE, "partition full"=FALSE, "last byte flushed"=FALSE}} ("element"), "datapath configs"=w286, "tagged llp packet"=w283, "output valid"=w284, "dram status"=w285) -> (w282:T27)
      }
      n95 = call "Create 4 In 4 Out Channel Resources.vi"("common resources"=w233) -> ("channel resources"=w259:T32)  [unwired: 14 in]
      n96 = Index Array(array=w254) -> (element #1=w213:T27, element #2=w214:T27, element #3=w215:T27, element #4=w217:T27)  [unwired: 4 in]
      n97 = Unbundle By Name(w259) -> ("so 0 resources"=w267:T29)
      n98 = Unbundle By Name(w213) -> ("output valid"=w253:bool, "tagged llp packet"=w252:T2, "datapath configs"=w251:T24, "dram status"=w250:T22)
      n99 = Unbundle By Name(w259) -> ("so 1 resources"=w268:T29)
      n100 = Unbundle By Name(w214) -> ("output valid"=w243:bool, "tagged llp packet"=w242:T2, "datapath configs"=w248:T24, "dram status"=w249:T22)
      n101 = Unbundle By Name(w259) -> ("so 2 resources"=w271:T29)
      n102 = Unbundle By Name(w215) -> ("output valid"=w245:bool, "tagged llp packet"=w244:T2, "datapath configs"=w247:T24, "dram status"=w246:T22)
      n103 = Unbundle By Name(w259) -> ("so 3 resources"=w270:T29)
      n104 = Unbundle By Name(w217) -> ("output valid"=w241:bool, "tagged llp packet"=w240:T2, "datapath configs"=w239:T24, "dram status"=w238:T22)
      n105 = Unbundle By Name(w213) -> ("datapath configs.enable i2c tap bridge"=w209:bool)
      n106 = Unbundle By Name(w214) -> ("datapath configs.enable i2c tap bridge"=w210:bool)
      n107 = Unbundle By Name(w215) -> ("datapath configs.enable i2c tap bridge"=w211:bool)
      n108 = Unbundle By Name(w217) -> ("datapath configs.enable i2c tap bridge"=w212:bool)
      n109 = Unbundle By Name(w259) -> ("si 0 resources.i2c io"=w229:T31, "so 0 resources.i2c io"=w219:T31)
      n110 = Unbundle By Name(w259) -> ("si 1 resources.i2c io"=w221:T31, "so 1 resources.i2c io"=w220:T31)
      n111 = Unbundle By Name(w259) -> ("si 2 resources.i2c io"=w222:T31, "so 2 resources.i2c io"=w218:T31)
      n112 = Unbundle By Name(w259) -> ("si 3 resources.i2c io"=w224:T31, "so 3 resources.i2c io"=w223:T31)
      n113 = call "Serial Output Channel Datapath.vi"("start trigger"=w279, "reset"=w216, "resources"=w268, "stop trigger"=w278, "generation counter"=w280, "output valid"=w243, "tagged llp packet"=w242, "configuration"=w248, "dram status"=w249) -> ("channel status"=w275:T26, "ready for start trigger"=w236:bool, "ready for input"=w269:bool)  [unwired: 4 in]
      n114 = call "Serial Output Channel Datapath.vi"("start trigger"=w279, "reset"=w216, "resources"=w267, "stop trigger"=w278, "generation counter"=w280, "output valid"=w253, "tagged llp packet"=w252, "configuration"=w251, "dram status"=w250) -> ("channel status"=w274:T26, "ready for start trigger"=w237:bool, "ready for input"=w266:bool)  [unwired: 4 in]
      n115 = call "Serial Output Channel Datapath.vi"("start trigger"=w279, "reset"=w216, "resources"=w271, "stop trigger"=w278, "generation counter"=w280, "output valid"=w245, "tagged llp packet"=w244, "configuration"=w247, "dram status"=w246) -> ("channel status"=w276:T26, "ready for start trigger"=w235:bool, "ready for input"=w272:bool)  [unwired: 4 in]
      n116 = call "Serial Output Channel Datapath.vi"("start trigger"=w279, "reset"=w216, "resources"=w270, "stop trigger"=w278, "generation counter"=w280, "output valid"=w241, "tagged llp packet"=w240, "configuration"=w239, "dram status"=w238) -> ("channel status"=w277:T26, "ready for start trigger"=w234:bool, "ready for input"=w273:bool)  [unwired: 4 in]
      n117 = call "I2C Tap Bridge.vi"("input channel i2c io"=w229, "reset"=w216, "output channel i2c io"=w219, "enable i2c tap bridge"=w209) -> ("i2c monitor"=w228:T23)  [unwired: 11 in]
      n118 = call "I2C Tap Bridge.vi"("input channel i2c io"=w221, "reset"=w216, "output channel i2c io"=w220, "enable i2c tap bridge"=w210) -> ("i2c monitor"=w225:T23)  [unwired: 11 in]
      n119 = call "I2C Tap Bridge.vi"("input channel i2c io"=w222, "reset"=w216, "output channel i2c io"=w218, "enable i2c tap bridge"=w211) -> ("i2c monitor"=w226:T23)  [unwired: 11 in]
      n120 = call "I2C Tap Bridge.vi"("input channel i2c io"=w224, "reset"=w216, "output channel i2c io"=w223, "enable i2c tap bridge"=w212) -> ("i2c monitor"=w227:T23)  [unwired: 11 in]
      n121 = Build Array(w274, w275, w276, w277) -> (w263:T26[])
      n122 = Build Array(w266, w269, w272, w273) -> (w230:bool[])
      n123 = for {
        tunnel: w263 -> [w290] mode=indexing
        tunnel: [w289] -> w265 mode=indexing
        n124 = Unbundle By Name(w290) -> ("packet timing error"=w289:bool)
      }
      n125 = for {
        tunnel: w263 -> [w288] mode=indexing
        tunnel: [w287] -> w262 mode=indexing
        n126 = Unbundle By Name(w288) -> ("generation done"=w287:bool)
      }
      n127 = Build Array(w237, w236, w235, w234) -> (w232:bool[])
      n128 = Build Array(w228, w225, w226, w227) -> (w260:T23[])
      n129 = And Array Elements(Boolean array=w232) -> (logical AND=w231:bool)
      n130 = And Array Elements(Boolean array=w262) -> (logical AND=w261:bool)
      n131 = Or Array Elements(Boolean array=w265) -> (logical OR=w264:bool)
    }
    frame condition #3 {
      # "Assert \"packet timing error detected\" if a \npacket timing error occurs on any channel."
      n132 = for {
        tunnel: w320 -> [w342] mode=indexing
        tunnel: w319 -> [w339] mode=indexing
        tunnel: w318 -> [w340] mode=indexing
        tunnel: w317 -> [w341] mode=indexing
        tunnel: [w338] -> w316 mode=indexing
        n133 = Bundle(cluster=T27 {"datapath configs"={"dram flush threshold (bytes)"=0, "packet data buffer fill threshold (bytes)"=0, "timestamp buffer fill threshold"=0, "packet timing error threshold (cycles)"=0, "channel enabled"=FALSE, "dram partition fill threshold (bytes)"=0, "enable i2c tap bridge"=FALSE, "packet timestamp offset (cycles)"=0}, "tagged llp packet"={"tag"={"timestamp"={"valid"=FALSE, "count"=0.0, "id"=enum."SI0 LLP", "metadata"=0}, "size"={"bytes"=0.0, "valid"=FALSE}}, "llp packet"={"header"={"word count"=0, "ecc"=0.0, "vcx"=0.0, "data type"=0.0, "vc"=0.0}, "header valid"=FALSE, "payload"={"end of payload"=FALSE, "end of payload index"=0.0, "payload data"=[]}, "payload valid"=FALSE, "footer"={"crc"=0}, "footer valid"=FALSE, "end of packet"=FALSE}}, "output valid"=FALSE, "dram status"={"bytes written"=0, "bytes read"=0, "overflow"=FALSE, "partition full"=FALSE, "last byte flushed"=FALSE}} ("element"), "datapath configs"=w342, "tagged llp packet"=w339, "output valid"=w340, "dram status"=w341) -> (w338:T27)
      }
      n134 = call "Create 4 In 4 Out Channel Resources.vi"("common resources"=w305) -> ("channel resources"=w321:T32)  [unwired: 14 in]
      n135 = Index Array(array=w316) -> (element #1=w293:T27, element #2=w294:T27)  [unwired: 2 in]
      n136 = Unbundle By Name(w321) -> ("so 0 resources"=w329:T29)
      n137 = Unbundle By Name(w293) -> ("output valid"=w315:bool, "tagged llp packet"=w314:T2, "datapath configs"=w313:T24, "dram status"=w312:T22)
      n138 = Unbundle By Name(w321) -> ("so 1 resources"=w330:T29)
      n139 = Unbundle By Name(w294) -> ("output valid"=w309:bool, "tagged llp packet"=w308:T2, "datapath configs"=w310:T24, "dram status"=w311:T22)
      n140 = Unbundle By Name(w293) -> ("datapath configs.enable i2c tap bridge"=w291:bool)
      n141 = Unbundle By Name(w294) -> ("datapath configs.enable i2c tap bridge"=w292:bool)
      n142 = Unbundle By Name(w321) -> ("si 0 resources.i2c io"=w301:T31, "so 0 resources.i2c io"=w296:T31)
      n143 = Unbundle By Name(w321) -> ("si 1 resources.i2c io"=w298:T31, "so 1 resources.i2c io"=w297:T31)
      n144 = call "Serial Output Channel Datapath.vi"("start trigger"=w335, "reset"=w295, "resources"=w330, "stop trigger"=w334, "generation counter"=w336, "output valid"=w309, "tagged llp packet"=w308, "configuration"=w310, "dram status"=w311) -> ("channel status"=w333:T26, "ready for start trigger"=w306:bool, "ready for input"=w331:bool)  [unwired: 4 in]
      n145 = call "Serial Output Channel Datapath.vi"("start trigger"=w335, "reset"=w295, "resources"=w329, "stop trigger"=w334, "generation counter"=w336, "output valid"=w315, "tagged llp packet"=w314, "configuration"=w313, "dram status"=w312) -> ("channel status"=w332:T26, "ready for start trigger"=w307:bool, "ready for input"=w328:bool)  [unwired: 4 in]
      n146 = call "I2C Tap Bridge.vi"("input channel i2c io"=w301, "reset"=w295, "output channel i2c io"=w296, "enable i2c tap bridge"=w291) -> ("i2c monitor"=w300:T23)  [unwired: 11 in]
      n147 = call "I2C Tap Bridge.vi"("input channel i2c io"=w298, "reset"=w295, "output channel i2c io"=w297, "enable i2c tap bridge"=w292) -> ("i2c monitor"=w299:T23)  [unwired: 11 in]
      n148 = Build Array(w332, w333) -> (w325:T26[])
      n149 = Build Array(w328, w331) -> (w302:bool[])
      n150 = for {
        tunnel: w325 -> [w346] mode=indexing
        tunnel: [w345] -> w327 mode=indexing
        n151 = Unbundle By Name(w346) -> ("packet timing error"=w345:bool)
      }
      n152 = for {
        tunnel: w325 -> [w344] mode=indexing
        tunnel: [w343] -> w324 mode=indexing
        n153 = Unbundle By Name(w344) -> ("generation done"=w343:bool)
      }
      n154 = Build Array(w307, w306) -> (w304:bool[])
      n155 = Build Array(w300, w299) -> (w322:T23[])
      n156 = And Array Elements(Boolean array=w304) -> (logical AND=w303:bool)
      n157 = And Array Elements(Boolean array=w324) -> (logical AND=w323:bool)
      n158 = Or Array Elements(Boolean array=w327) -> (logical OR=w326:bool)
    }
    frame condition #4 (active) {
      w347 = TRUE ("assert")
      # "Target not supported"
      n159 = call <instrlib>:"Assert.vi"("assert"=w347, "error code"=-1, "enable show error"=w347) -> ()  [unwired: 13 in]
    }
  }
  "serial output channel status" <- w12
  "ready for start trigger" <- w4
  "packet timing error detected" <- w13
  "generation done" <- w11
  "i2c monitor array" <- w10
  "ready for input" <- w3
